vi "Globals - Monitoring Variables.vi"() -> ()   [LabVIEW 2013]
panel:
  in  "Send Live Data":bool
  in  "Live Data Channel":u32
  in  "Drive Space":dbl
  in  "Buffer Backlog":dbl
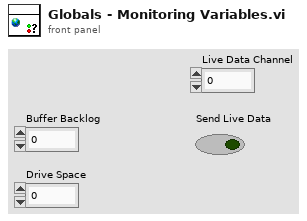
[diagram p1: front panel]
diagram:
